vi "RPC Get Fault Log.vi"(6 "timeout (s)":dbl=60.0 format="%#_13g", 8 "error in (no error)":errorcluster, 10 "index":u8, 11 "BLE address in":string) -> (0 "error out":errorcluster, 1 "info":string, 2 "nth":u32, 3 "BLE address out":string, 4 "has log?":bool)   [LabVIEW 2017]
uses:
  <vilib>/addons/InsightCM/Utilities/BleBackdoor/RPC Commands.ctl
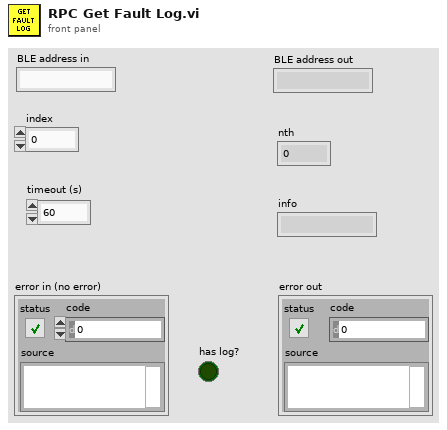
[diagram p1: front panel]
types:
  T1 = typedef "RPC Commands.ctl" = u16
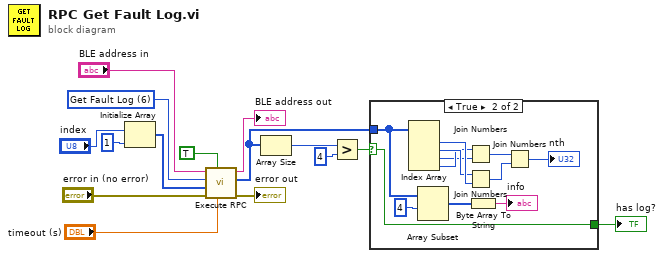
[diagram p0: block diagram]
diagram:
  w10 = T1 6 items=["Debug Print", "Configure ATECC", "Set Signed Identity", "Erase Bonds and Power Off", "Get Spider Cal Constants", "Get Reset Reason", "Get Fault Log", "Set Mac Address"] ("RPC Command")
  n1 = Initialize Array("index", 1 ("dimension size")) -> (w7:u8[])
  n2 = call <vilib>:"Execute RPC.vi"("timeout (s)"="timeout (s)", "encrypt (false)"=TRUE, "error in (no error)"="error in (no error)", "request"=w7, "RPC Command"=w10, "target endpoint MAC address in"="BLE address in") -> ("error out"=→"error out":errorcluster, "response"=w2:u8[], "target endpoint MAC address out"=→"BLE address out":string)  [unwired: 3 in]
  n3 = Array Size(array=w2) -> (size(s)=w6:i32)
  n4 = Greater?(x=w6, y=4) -> (0:w4:bool)
  n5 = case shown="True" w4 {
    selector: w4 -> [w16 w28]
    tunnel: [w16 w28] -> w3
    tunnel: w2 -> [_ w20]
    frame False {
    }
    frame True {
      n6 = Index Array(array=w20) -> (element #1=w27:u8, element #2=w26:u8, element #3=w24:u8, element #4=w25:u8)  [unwired: 4 in]
      n7 = Array Subset(array=w20, index=4) -> (w18:u8[])  [unwired: 1 in]
      n8 = Join Numbers(hi=w25, lo=w24) -> ((hi.lo)=w21:u16)
      n9 = Join Numbers(hi=w26, lo=w27) -> ((hi.lo)=w22:u16)
      n10 = Byte Array To String(unsigned byte array=w18) -> (string=→"info":string)
      n11 = Join Numbers(hi=w21, lo=w22) -> ((hi.lo)=→"nth":u32)
    }
  }
  "has log?" <- w3
